vi "Config Spark Max Output HW Get Set.vi"(6 "Get(f) Set(t)":bool, 7 "SparkMax Output":T1, 8 "Error":errorcluster, 11 "Drive Refs":T3) -> (0 "Error Out":errorcluster, 3 "Drive Refs Out":T3, 5 "SparkMax Output Out":T1)   [LabVIEW 2020, in "Swerve AM_ACT.lvlib"]
uses:
  Swerve AM_ACT.lvlib
  <vilib>/Rock Robotics/WPI/MotorControl/WPI_MotorControlDeviceRef.ctl
  <vilib>/Rock Robotics/WPI/MotorControl/WPI_MotorControlType.ctl
  <vilib>/Rock Robotics/SystemInterfaces/DIO/FPGA_DIOPWMChannel.ctl
  <vilib>/Rock Robotics/WPI/PWM/WPI_PWMDeadband.ctl
  <vilib>/Rock Robotics/SystemInterfaces/DIO/FPGA_DIOChannel.ctl
  Shared Code/TypeDefs/Cluster_Config Spark Max Motor Output.ctl
  <vilib>/Rock Robotics/WPI/ThirdParty/REV Robotics/REVLib/Typedef/Spark MAX Idle Mode.ctl
  <vilib>/Utility/Data Type/NI_Data Type.lvlib
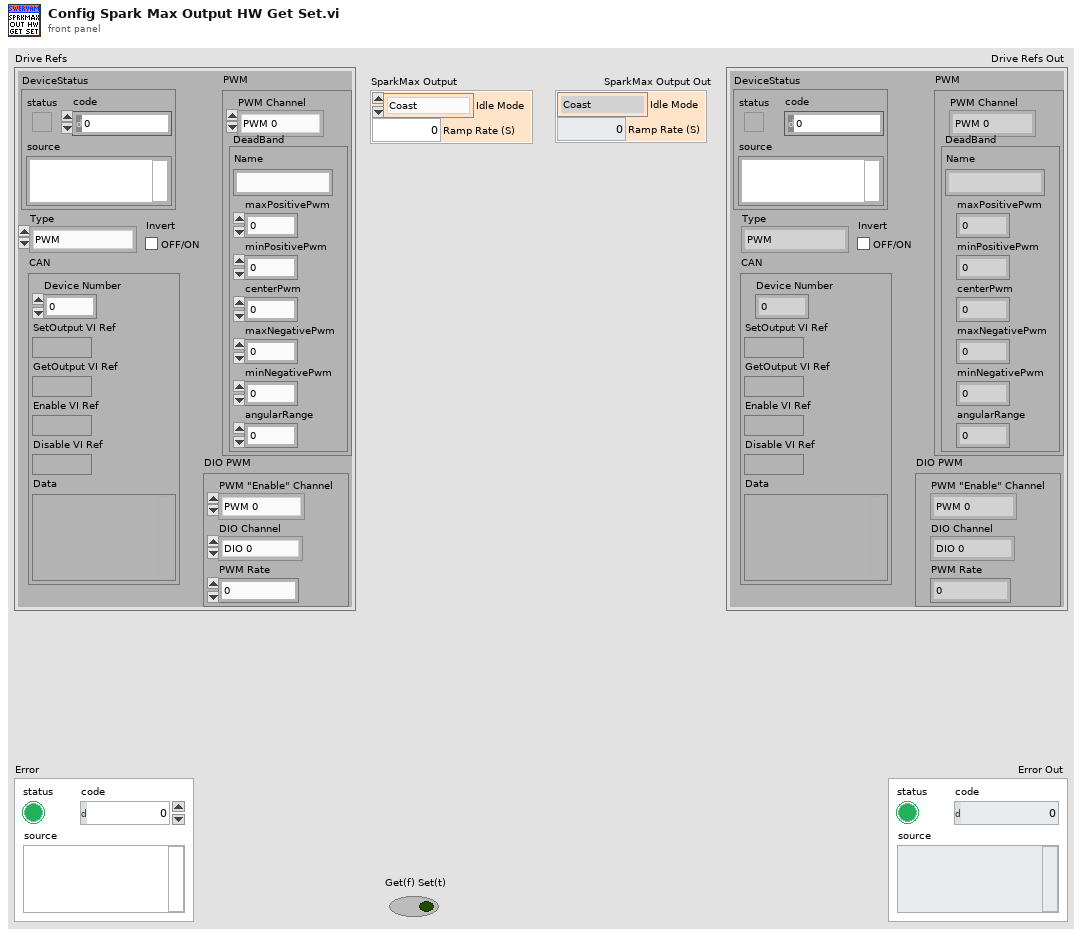
[diagram p1: front panel]
types:
  T1 = typedef "Cluster_Config Spark Max Motor Output.ctl" = cluster{"Idle Mode":T2, "Ramp Rate (S)":dbl}
  T2 = typedef "Spark MAX Idle Mode.ctl" = enum16{"Coast", "Brake"}
  T3 = typedef "WPI_MotorControlDeviceRef.ctl" = cluster{"DeviceStatus":errorcluster, "Type":T4, "PWM":cluster{"PWM Channel":T5, "DeadBand":T6}, "CAN":cluster{"Device Number":u8, "SetOutput VI Ref":variant, "GetOutput VI Ref":variant, "Enable VI Ref":variant, "Disable VI Ref":variant, "Data":variant}, "Invert":bool, "DIO PWM":cluster{"PWM \"Enable\" Channel":T5, "DIOChannel":T7, "PWM Rate":dbl}}
  T4 = typedef "WPI_MotorControlType.ctl" = enum16{"PWM", "CAN", "DIO PWM"}
  T5 = typedef "FPGA_DIOPWMChannel.ctl" = enum8{"PWM 0", "PWM 1", "PWM 2", "PWM 3", "PWM 4", "PWM 5", "PWM 6", "PWM 7", "PWM 8", "PWM 9", "PWM MXP 0", "PWM MXP 1", "PWM MXP 2", "PWM MXP 3", "PWM MXP 4", "PWM MXP 5", "PWM MXP 6", "PWM MXP 7", "PWM MXP 8", "PWM MXP 9", "Invalid"}
  T6 = typedef "WPI_PWMDeadband.ctl" = cluster{"Name":string, "maxPositivePwm":i32, "minPositivePwm":i32, "centerPwm":i32, "maxNegativePwm":i32, "minNegativePwm":i32, "angularRange":u16}
  T7 = typedef "FPGA_DIOChannel.ctl" = enum8{"DIO 0", "DIO 1", "DIO 2", "DIO 3", "DIO 4", "DIO 5", "DIO 6", "DIO 7", "DIO 8", "DIO 9", "DIO MXP 0", "DIO MXP 1", "DIO MXP 2", "DIO MXP 3", "DIO MXP 4", "DIO MXP 5", "DIO MXP 6", "DIO MXP 7", "DIO MXP 8", "DIO MXP 9", "DIO MXP 10", "DIO MXP 11", "DIO MXP 12", "DIO MXP 13", "DIO MXP 14", "DIO MXP 15", "SPI Port CS1", "SPI Port CS2", "SPI Port CS3", "SPI Port MISO", "SPI Port MOSI", "Invalid"}
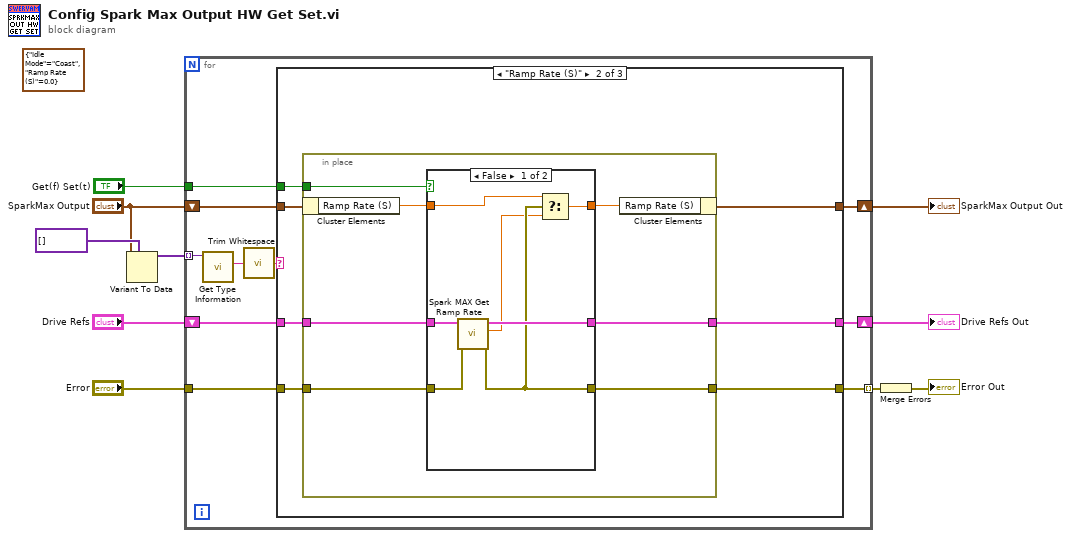
[diagram p0: block diagram]
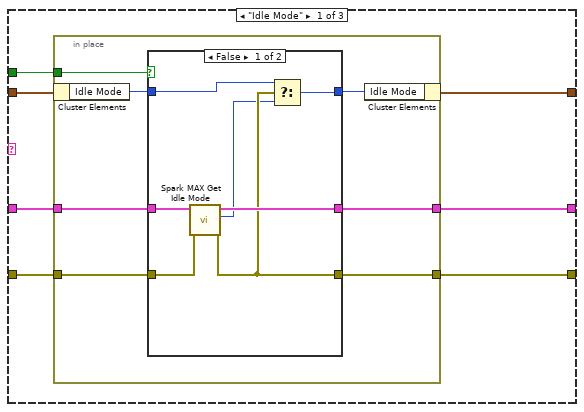
[diagram p2: hidden frame]
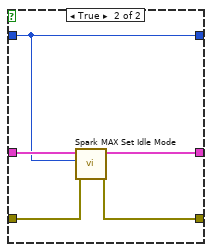
[diagram p3: hidden frame]
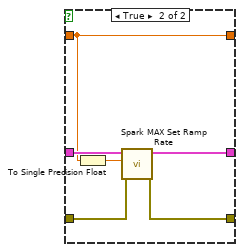
[diagram p4: hidden frame]
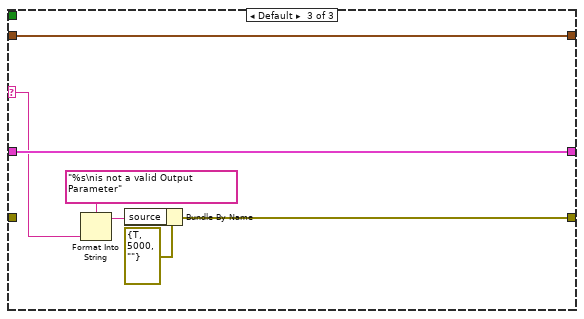
[diagram p5: hidden frame]
diagram:
  (unwired) T1 {"Idle Mode"=enum."Coast", "Ramp Rate (S)"=0.0} ("SparkMax Output")
  n1 = Variant To Data(type=variant[] [], Variant="SparkMax Output") -> (data=w5:variant[])  [unwired: 1 in, 1 out]
  n2 = for {
    shift-right: [w11] -> w10
    shift-left: "SparkMax Output" -> [w17]
    shift-right: [w12] -> w8
    shift-left: "Drive Refs" -> [w16]
    tunnel: "Get(f) Set(t)" -> [w15]
    tunnel: w5 -> [w19] mode=indexing
    tunnel: "Error" -> [w14]
    tunnel: [w13] -> w2 mode=indexing
    n3 = call <vilib>:"Get Type Information.vi"("variant"=w19) -> ("name"=w20:string)  [unwired: 6 in, 4 out]
    n4 = call <vilib>:"Trim Whitespace.vi"("string"=w20) -> ("trimmed string"=w18:string)  [unwired: 1 in]
    n5 = case shown="\"Ramp Rate (S)\"" w18 {
      selector: w18 -> [_ _ w78]
      tunnel: w17 -> [w27 w53 w80]
      tunnel: w16 -> [w23 w49 w79]
      tunnel: w15 -> [w26 w52 _]
      tunnel: w14 -> [w25 w51 _]
      tunnel: [w24 w50 w76] -> w13
      tunnel: [w22 w48 w79] -> w12
      tunnel: [w21 w47 w80] -> w11
      frame "Idle Mode" {
        n6 = in-place {
          in-place-border: w26 -> [w34]
          in-place-border: w25 -> [w32]
          in-place-border: [w31] -> w24
          in-place-border: w23 -> [w30]
          in-place-border: [w29] -> w22
          n7 = in-place-cluster #1(w27) -> ("Idle Mode"=w33:T2)
          n8 = case shown="False" w34 {
            tunnel: w33 -> [w37 w44]
            tunnel: w32 -> [w39 w42]
            tunnel: [w38 w43] -> w31
            tunnel: w30 -> [w41 w46]
            tunnel: [w40 w45] -> w29
            tunnel: [w35 w44] -> w28
            frame False {
              n9 = call <vilib>:"Spark MAX Get Idle Mode.vi"("error in (no error)"=w39, "MotorControlDeviceRef in"=w41) -> ("error out"=w38:errorcluster, "Idle Mode"=w36:T2, "MotorControlDeviceRef out"=w40:T3)  [unwired: 7 in]
              n10 = Select(t=w37, s=w38, f=w36) -> (s? t:f=w35:T2)
            }
            frame True {
              n11 = call <vilib>:"Spark MAX Set Idle Mode.vi"("error in (no error)"=w42, "Idle Mode"=w44, "MotorControlDeviceRef in"=w46) -> ("error out"=w43:errorcluster, "MotorControlDeviceRef out"=w45:T3)  [unwired: 7 in]
            }
          }
          n12 = in-place-cluster #1("Idle Mode"=w28) -> (w21:T1)
        }
      }
      frame "Ramp Rate (S)" {
        n13 = in-place {
          in-place-border: w52 -> [w60]
          in-place-border: w51 -> [w58]
          in-place-border: [w57] -> w50
          in-place-border: w49 -> [w56]
          in-place-border: [w55] -> w48
          n14 = in-place-cluster #2(w53) -> ("Ramp Rate (S)"=w59:dbl)
          n15 = case shown="False" w60 {
            tunnel: w59 -> [w63 w71]
            tunnel: w58 -> [w65 w69]
            tunnel: [w64 w70] -> w57
            tunnel: w56 -> [w67 w73]
            tunnel: [w66 w72] -> w55
            tunnel: [w61 w71] -> w54
            frame False {
              n16 = call <vilib>:"Spark MAX Get Ramp Rate.vi"("error in (no error)"=w65, "MotorControlDeviceRef in"=w67) -> ("error out"=w64:errorcluster, "Ramp Rate"=w62:dbl, "MotorControlDeviceRef out"=w66:T3)  [unwired: 7 in]
              n17 = Select(t=w63, s=w64, f=w62) -> (s? t:f=w61:dbl)
            }
            frame True {
              n18 = To Single Precision Float(number=w71) -> (single precision float=w68:sgl)
              n19 = call <vilib>:"Spark MAX Set Ramp Rate.vi"("error in (no error)"=w69, "Seconds from neutral to full (0)"=w68, "MotorControlDeviceRef in"=w73) -> ("error out"=w70:errorcluster, "MotorControlDeviceRef"=w72:T3)  [unwired: 7 in]
            }
          }
          n20 = in-place-cluster #2("Ramp Rate (S)"=w54) -> (w47:T1)
        }
      }
      frame Default {
        n21 = Format Into String(format string="%s\nis not a valid Output Parameter", w78) -> (resulting string=w74:string)  [unwired: 2 in, 1 out]
        n22 = Bundle By Name(cluster=errorcluster {"status"=TRUE, "code"=5000, "source"=""} ("error out"), "source"=w74) -> (w76:errorcluster)
      }
    }
  }
  "Drive Refs Out" <- w8
  "SparkMax Output Out" <- w10
  n23 = Merge Errors(w2) -> (→"Error Out":errorcluster)
